vi "runtime io test.vi"() -> ()   [LabVIEW 2013, in "CVT tests.lvlib"]
uses:
  CVT tests.lvlib
  <vilib>/NI/Tag Bus Module Framework/channel/channel classification.ctl
  execution/CVT runtime.lvclass
  configuration/CVT configuration.lvclass
  <vilib>/NI/Tag Bus Module Framework/root configuration/TBM configuration.lvclass/TBM configuration.ctl
  <vilib>/NI/Tag Bus/tag/tag descriptor.lvclass/tag descriptor.ctl
  configuration/CVT configuration.lvclass/CVT configuration.ctl
  <vilib>/NI/Tag Bus/table/data polymorphs/write one/write Double.vi
  <vilib>/NI/Tag Bus/table/data polymorphs/read one/read Double.vi
  <vilib>/NI/Tag Bus Module Framework/root configuration/Read instance name.vi
  configuration/Write channels.vi
  <vilib>/NI/Tag Bus/tag/read tag name.vi
  <vilib>/NI/Tag Bus/tag/read data type.vi
  <vilib>/NI/Tag Bus Module Framework/channel/TBM channel.lvclass
  <vilib>/NI/Tag Bus Module Framework/root configuration/TBM configuration.lvclass
  <vilib>/NI/Tag Bus/dictionary/data dictionary.lvclass
  <vilib>/NI/Tag Bus/table/data table.lvlib
panel:
  out "inputs changed?":bool
  out "no error":errorcluster
  # "This is expected to remain false until you write code for input"
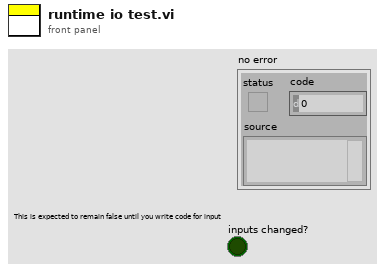
[diagram p1: front panel]
types:
  T1 = typedef "TBM channel.lvclass/channel classification.ctl" = enum16{"input data", "output data", "processing parameter", "processing result"}
  T2 = typedef "tag bus.lvlib/tag descriptor.lvclass/Data Type.ctl" = enum16{"Double", "Single", "I64", "I32", "I16", "I8", "U64", "U32", "U16", "U8", "Boolean", "String", "Array of Double", "Array of Single", "Array of I64", "Array of I32", "Array of I16", "Array of I8", "Array of U64", "Array of U32", "Array of U16", "Array of U8", "Array of Boolean", "Array of String"}
  T3 = typedef "TBM channel.lvclass/data tables.ctl" = cluster{"input data":T4, "processing parameter":T4, "processing result":T4, "output data":T4}
  T4 = typedef "tag bus.lvlib/dictionary table pair.ctl" = cluster{"data dictionary":refnum<class "data dictionary.lvclass">, "data table":T5}
  T5 = typedef "tag bus.lvlib/data table.lvlib/data table.ctl" = cluster{"Double":dbl[], "Single":sgl[], "I64":i64[], "I32":i32[], "I16":i16[], "I8":i8[], "U64":u64[], "U32":u32[], "U16":u16[], "U8":u8[], "Boolean":bool[], "String":string[], "Array of Double":cluster{"DBL Array":dbl[]}[], "Array of Single":cluster{"SGL Array":sgl[]}[], "Array of I64":cluster{"I64 Array":i64[]}[], "Array of I32":cluster{"I32 Array":i32[]}[], "Array of I16":cluster{"I16 Array":i16[]}[], "Array of I8":cluster{"I8 Array":i8[]}[], "Array of U64":cluster{"U64 Array":u64[]}[], "Array of U32":cluster{"U32 Array":u32[]}[], "Array of U16":cluster{"U16 Array":u16[]}[], "Array of U8":cluster{"U8 Array":u8[]}[], "Array of Boolean":cluster{"Boolean Array":bool[]}[], "Array of String":cluster{"String Array":string[]}[]}
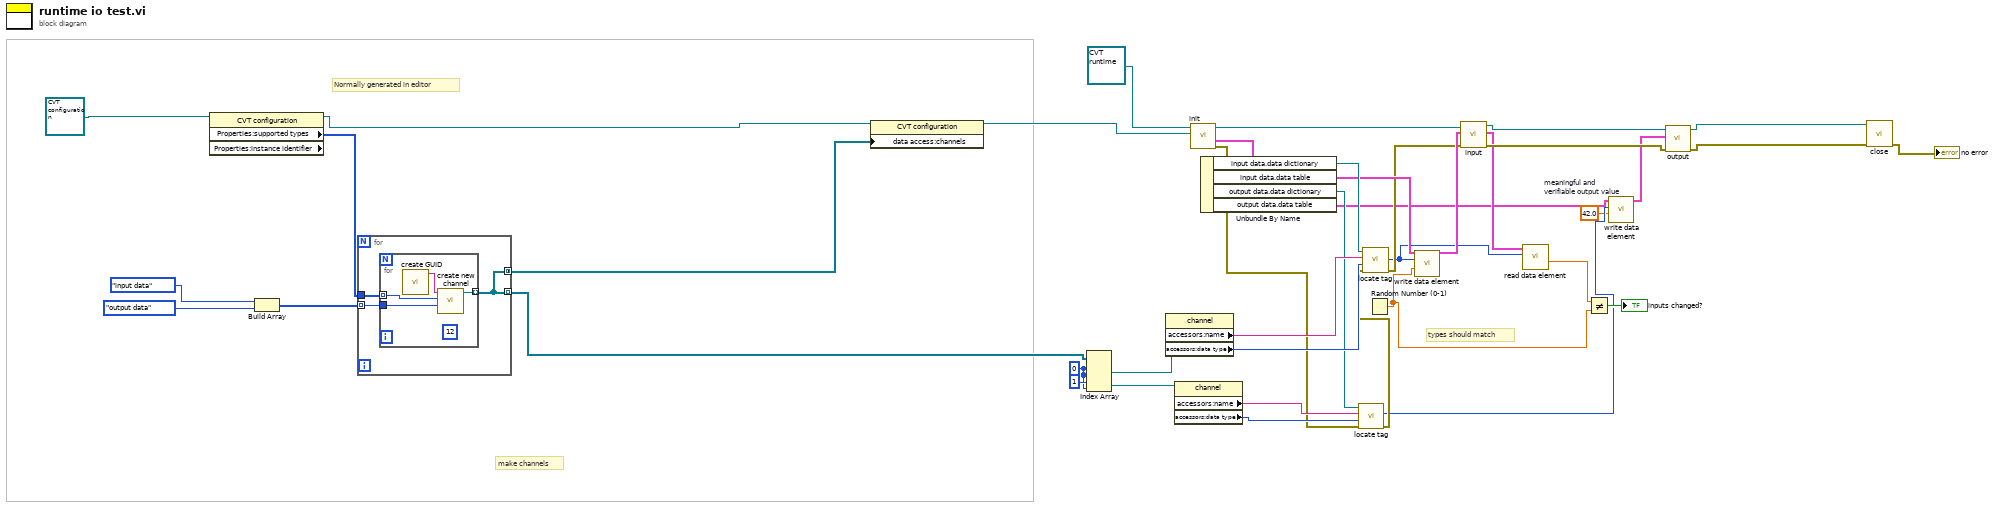
[diagram p0: block diagram]
diagram:
  w6 = 42.0  # meaningful and verifiable output value
  w35 = 0 ("index (row)")
  # "types should match"
  # "Normally generated in editor"
  # "make channels"
  n1 = property class="CVT configuration" props=["Properties:supported types", "Properties:instance identifier"](reference=refnum<class "CVT configuration.lvclass"> refnum ("tag bus configurable plugin module configuration")) -> (reference out=w1:refnum<class "CVT configuration.lvclass">, "Properties:supported types"=w38:T2[])  [unwired: 1 in, 2 out]
  n2 = Build Array(channel_classification."input data" ("channel classification"), channel_classification."output data" ("channel classification")) -> (w39:T1[])
  n3 = for {
    tunnel: w39 -> [w44] mode=indexing
    tunnel: [w42] -> w37 mode=indexing
    tunnel: w38 -> [w43]
    tunnel: [w42] -> w2 mode=concatenating
    n4 = for {
      tunnel: w44 -> [w47]
      tunnel: [w48] -> w42 mode=indexing
      tunnel: w43 -> [w46] mode=indexing
      (unwired) 12
      n5 = call <vilib>:"create GUID.vi"() -> ("uuid"=w45:string)  [unwired: 11 in]
      n6 = call <vilib>:"create new channel.vi"("channel classification"=w47, "data type"=w46, "channel name"=w45) -> ("channel"=w48:refnum<class "TBM channel.lvclass">)  [unwired: 8 in]
    }
  }
  n7 = property class="CVT configuration"(reference=w1, "data access:channels"=w2) -> (reference out=w3:refnum<class "CVT configuration.lvclass">)  [unwired: 1 in, 1 out]
  n8 = Index Array(array=w37, index (row) #1=w35, index (col) #1=w35, index (row) #2=1 ("index (row)"), index (col) #2=w35) -> (element #1=w26:refnum<class "TBM channel.lvclass">, element #2=w15:refnum<class "TBM channel.lvclass">)
  n9 = property class="channel"(reference=w26) -> ("accessors:name"=w24:string, "accessors:data type"=w25:T2)  [unwired: 1 in, 2 out]
  n10 = property class="channel"(reference=w15) -> ("accessors:name"=w13:string, "accessors:data type"=w12:T2)  [unwired: 1 in, 2 out]
  n11 = call-dynamic "init.vi"("TBM module configuration in"=w3, "CVT runtime in"=refnum<class "CVT runtime.lvclass"> refnum ("tag bus configurable plugin module")) -> ("error out"=w11:errorcluster, "data allocations"=w28:T3, "CVT runtime out"=w29:refnum<class "CVT runtime.lvclass">)  [unwired: 6 in, 1 out]
  n12 = Unbundle By Name(w28) -> ("input data.data dictionary"=w27:refnum<class "data dictionary.lvclass">, "input data.data table"=w23:T5, "output data.data dictionary"=w14:refnum<class "data dictionary.lvclass">, "output data.data table"=w9:T5)
  n13 = call <vilib>:"locate tag.vi"("error in"=w11, "data type"=w12, "name"=w13, "data dictionary in"=w14) -> ("error out"=w10:errorcluster, "index"=w7:i32)  [unwired: 5 in, 1 out]
  n14 = call <vilib>:"locate tag.vi"("error in"=w10, "data type"=w25, "name"=w24, "data dictionary in"=w27) -> ("error out"=w21:errorcluster, "index"=w19:i32)  [unwired: 5 in, 1 out]
  n15 = Random Number (0-1)() -> (number: 0 to 1=w18:dbl)
  n16 = call-poly <vilib>:"write data element.vi"("value"=w18, "index"=w19, "data table in"=w23) -> ("data table out"=w22:T5)  [unwired: 8 in]
  n17 = call-dynamic "input.vi"("error in"=w21, "data table in"=w22, "CVT runtime in"=w29) -> ("error out"=w30:errorcluster, "data table out"=w20:T5, "CVT runtime out"=w31:refnum<class "CVT runtime.lvclass">)  [unwired: 6 in]
  n18 = call-poly <vilib>:"read data element.vi"("index"=w19, "data table in"=w20) -> ("value"=w17:dbl)  [unwired: 8 in, 1 out]
  n19 = Not Equal?(x=w17, y=w18) -> (x != y?=→"inputs changed?":bool)
  n20 = call-poly <vilib>:"write data element.vi"("value"=w6, "index"=w7, "data table in"=w9) -> ("data table out"=w8:T5)  [unwired: 8 in]
  n21 = call-dynamic "output.vi"("error in"=w30, "data table in"=w8, "CVT runtime in"=w31) -> ("error out"=w32:errorcluster, "CVT runtime out"=w33:refnum<class "CVT runtime.lvclass">)  [unwired: 6 in, 1 out]
  n22 = call-dynamic "close.vi"("error in"=w32, "CVT runtime in"=w33) -> ("error out"=→"no error":errorcluster)  [unwired: 9 in]
